vi "REF_EDITOR_by_station_name.vi"(7 "actual_reference_name":string, 10 "records_input":string[][](array[string])) -> (3 "records_output":string[][](array[string]))   [LabVIEW 2020]
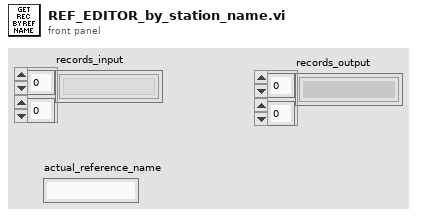
[diagram p1: front panel]
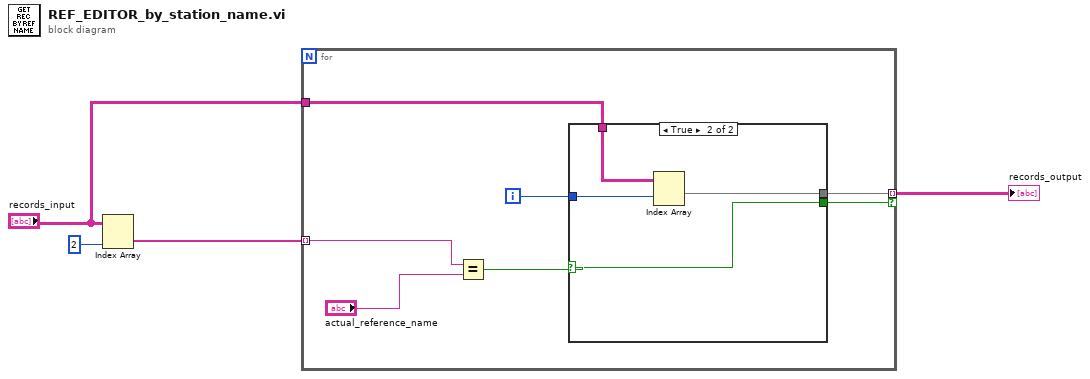
[diagram p0: block diagram]
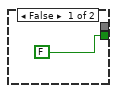
[diagram p2: hidden frame]
diagram:
  n1 = Index Array(array="records_input", index (col)=2) -> (element=w3:string[])  [unwired: 1 in]
  n2 = for {
    tunnel: w3 -> [w10] mode=indexing
    tunnel: "records_input" -> [w7]
    tunnel: [w6] -> w1 mode=indexing if=w5
    i -> [w8]
    n3 = Equal?(x=w10, y="actual_reference_name") -> (x = y?=w9:bool)
    n4 = case shown="True" w9 {
      selector: w9 -> [_ w14]
      tunnel: w7 -> [_ w16]
      tunnel: w8 -> [_ w13]
      tunnel: [_ w15] -> w6
      tunnel: [FALSE w14] -> w5
      frame False {
      }
      frame True {
        n5 = Index Array(array=w16, index (row)=w13) -> (element=w15:string[])  [unwired: 1 in]
      }
    }
  }
  "records_output" <- w1
